vi "MessageName.vi"() -> (2 "MessageName":string)   [LabVIEW 2020, in "PB Msg Template.lvlib"]
uses:
  PB Msg Template.lvlib
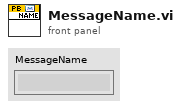
[diagram p1: front panel]
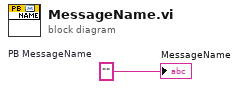
[diagram p0: block diagram]
diagram:
  w1 = ""  # PB MessageName
  "MessageName" <- w1
